vi "select spot to track.vi"(10 "new circle":bool, 11 "N spot tracker in":T1) -> (1 "use photons to track":bool, 3 "N spot tracker out":T1)   [LabVIEW 2010]
uses:
  kalman N spot state.ctl
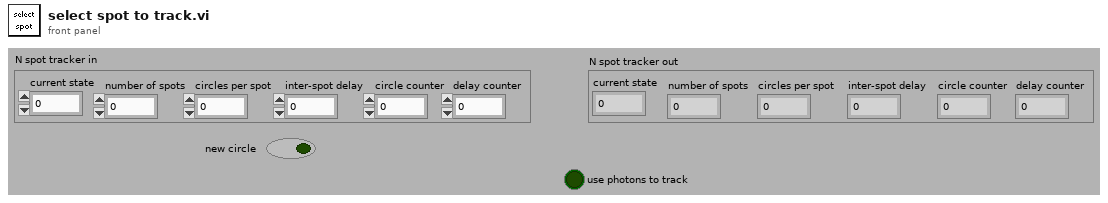
[diagram p1: front panel]
types:
  T1 = typedef "kalman N spot state.ctl" = cluster{"current state":u8, "number of spots":u8, "circles per spot":u16, "inter-spot delay":u8, "circle counter":u16, "delay counter":u8}
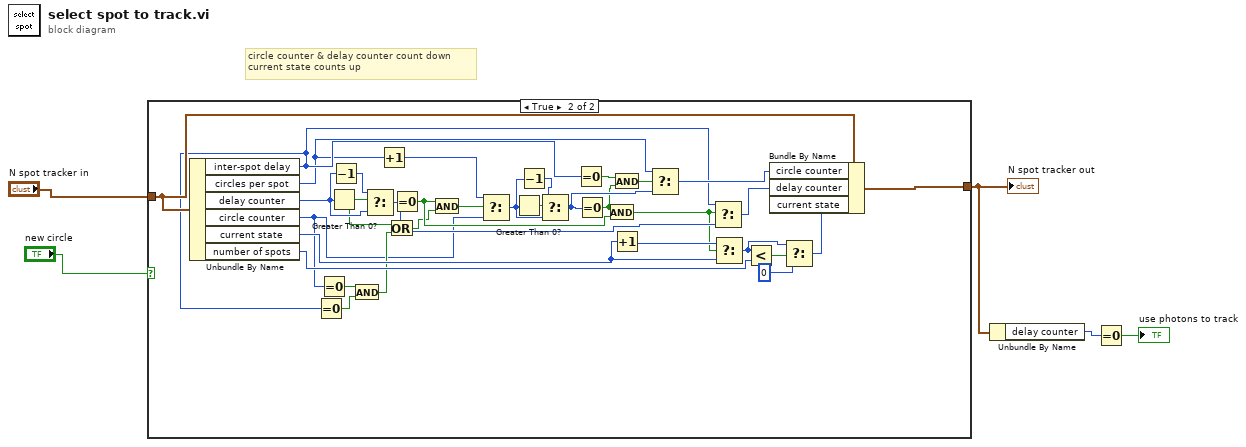
[diagram p0: block diagram]
diagram:
  # "circle counter & delay counter count down\ncurrent state counts up"
  n1 = case shown="True" "new circle" {
    tunnel: "N spot tracker in" -> [w6 w24]
    tunnel: [w6 w25] -> w1
    frame False {
    }
    frame True {
      n2 = Unbundle By Name(w24) -> ("inter-spot delay"=w11:u8, "circles per spot"=w10:u16, "delay counter"=w23:u8, "circle counter"=w14:u16, "current state"=w32:u8, "number of spots"=w31:u8)
      n3 = Equal To 0?(x=w11) -> (x = 0?=w17:bool)
      n4 = Equal To 0?(x=w14) -> (x = 0?=w18:bool)
      n5 = Greater Than 0?(x=w23) -> (x > 0?=w19:bool)
      n6 = Decrement(x=w23) -> (x-1=w39:u8)
      n7 = And(x=w18, y=w17) -> (x .and. y?=w15:bool)
      n8 = Select(t=w39, s=w19, f=w23) -> (s? t:f=w34:u8)
      n9 = Increment(x=w10) -> (x+1=w20:u16)
      n10 = Or(x=w19, y=w15) -> (x .or. y?=w16:bool)
      n11 = Equal To 0?(x=w34) -> (x = 0?=w21:bool)
      n12 = And(x=w21, y=w16) -> (x .and. y?=w38:bool)
      n13 = Select(t=w20, s=w38, f=w14) -> (s? t:f=w36:u16)
      n14 = Greater Than 0?(x=w36) -> (x > 0?=w35:bool)
      n15 = Decrement(x=w36) -> (x-1=w37:u16)
      n16 = Select(t=w37, s=w35, f=w36) -> (s? t:f=w12:u16)
      n17 = Equal To 0?(x=w11) -> (x = 0?=w8:bool)
      n18 = Equal To 0?(x=w12) -> (x = 0?=w7:bool)
      n19 = And(x=w7, y=w21) -> (x .and. y?=w22:bool)
      n20 = And(x=w8, y=w7) -> (x .and. y?=w9:bool)
      n21 = Increment(x=w32) -> (x+1=w33:u8)
      n22 = Select(t=w10, s=w9, f=w12) -> (s? t:f=w13:u16)
      n23 = Select(t=w11, s=w22, f=w34) -> (s? t:f=w26:u8)
      n24 = Select(t=w33, s=w22, f=w32) -> (s? t:f=w29:u8)
      n25 = Less?(x=w29, y=w31) -> (x < y?=w30:bool)
      n26 = Select(t=w29, s=w30, f=u8 0) -> (s? t:f=w27:u8)
      n27 = Bundle By Name(cluster=w24, "circle counter"=w13, "delay counter"=w26, "current state"=w27) -> (w25:T1)
    }
  }
  "N spot tracker out" <- w1
  n28 = Unbundle By Name(w1) -> ("delay counter"=w2:u8)
  n29 = Equal To 0?(x=w2) -> (x = 0?=→"use photons to track":bool)
